vi "Create Ribbon.vi"(6 "Draw Mode":T7(ring)=enum."Triangles", 7 "3D Ribbon Property":T1={"General Property"={"Plot Name"="", "Coordinate System"=enum."Cartesian", "Opacity"=0.0}, "Projection Property"={"Draw XY"=FALSE, "Draw YZ"=FALSE, "Draw XZ"=FALSE}, "Plot Property"={"Draw Surface"=FALSE, "Color Ramp Cluster"={"Color Ramp Style"=enum."None", "Color Ramp Array"=[16711934, 393471, 57855, 4390754, 16449346, 16744722, 16711680], "Color Ramp Index"=[45, 91, 133, 175, 219, 255], "Interpolate?"=FALSE, "Logarithm?"=FALSE}, "Line Style"=enum."None", "Line Width"=0.0, "Line Color"=0, "Antialiasing"=FALSE}, "Ribbon Property"={"Ribbon Mode"=enum."Row", "Ribbon Width"=0.0}}, 8 "error in (no error)":errorcluster, 10 "Plot Representation In":T4, 11 "Plot Object In":refnum<vi>) -> (0 "error out":errorcluster, 2 "Plot Representation Out":T4, 3 "Plot Object Out":refnum<vi>, 4 "Ribbon Object Out":refnum<vi>)   [LabVIEW 2020, in "3D Ribbon.lvclass"]
uses:
  <vilib>/Math Plots/3D Math Plots/3D Ribbon/3D Ribbon/3D Ribbon.lvclass
  <vilib>/Math Plots/3D Math Plots/3D Plot/3D Plot/Typedef/Plot Representation.ctl
  <vilib>/Math Plots/3D Math Plots/3D Plot/3D Plot/Typedef/Range Clusters.ctl
  <vilib>/Math Plots/3D Math Plots/3D Plot/3D Plot/Typedef/Mesh Data.ctl
  <vilib>/Math Plots/3D Math Plots/3D Ribbon/3D Ribbon/Typedef/3D Ribbon Property.ctl
  <vilib>/Math Plots/3D Math Plots/3D Plot/3D Plot/Typedef/Color Ramp Cluster.ctl
  <vilib>/Math Plots/3D Math Plots/3D Plot/3D Plot/Typedef/Line Type.ctl
  <vilib>/picture/3D Picture Control/NI_3D Picture Control.lvlib
  <vilib>/Math Plots/3D Math Plots/3D Plot/3D Plot/3D Plot.lvclass
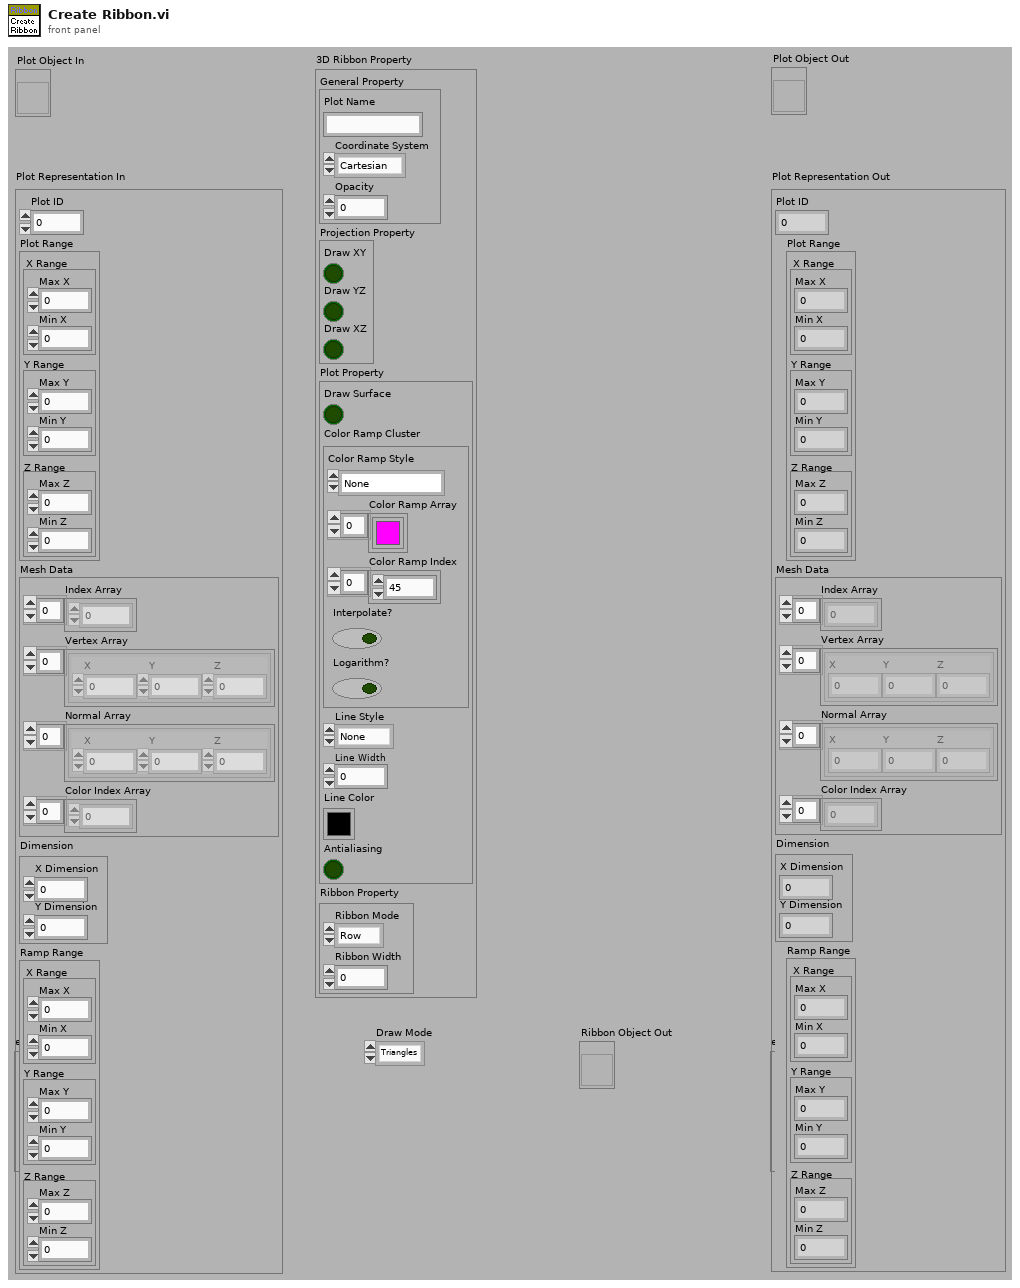
[diagram p1: front panel]
types:
  T1 = typedef "3D Ribbon.lvclass/3D Ribbon Property.ctl" = cluster{"General Property":cluster{"Plot Name":string, "Coordinate System":enum16{"Cartesian", "Cylindrical", "Spherical"}, "Opacity":sgl}, "Projection Property":cluster{"Draw XY":bool, "Draw YZ":bool, "Draw XZ":bool}, "Plot Property":cluster{"Draw Surface":bool, "Color Ramp Cluster":T2, "Line Style":T3, "Line Width":sgl, "Line Color":u32, "Antialiasing":bool}, "Ribbon Property":cluster{"Ribbon Mode":enum16{"Row", "Column"}, "Ribbon Width":sgl}}
  T2 = typedef "3D Plot.lvclass/Color Ramp Cluster.ctl" = cluster{"Color Ramp Style":enum16{"None", "Shaded", "Color spectrum", "Grey scale", "Custom"}, "Color Ramp Array":u32[], "Color Ramp Index":i32[], "Interpolate?":bool, "Logarithm?":bool}
  T3 = typedef "3D Plot.lvclass/Line Type.ctl" = enum16{"None", "Solid", "Dash", "Dot", "Dash Dot"}
  T4 = typedef "3D Plot.lvclass/Plot Representation.ctl" = cluster{"Plot ID":i32, "Plot Range":T5, "Mesh Data":T6, "Dimension":cluster{"X Dimension":i32, "Y Dimension":i32}, "Ramp Range":T5}
  T5 = typedef "3D Plot.lvclass/Range Clusters.ctl" = cluster{"X Range":cluster{"Max X":sgl, "Min X":sgl}, "Y Range":cluster{"Max Y":sgl, "Min Y":sgl}, "Z Range":cluster{"Max Z":sgl, "Min Z":sgl}}
  T6 = typedef "3D Plot.lvclass/Mesh Data.ctl" = cluster{"Index Array":u32[], "Vertex Array":cluster{"X":sgl, "Y":sgl, "Z":sgl}[], "Normal Array":cluster{"X":sgl, "Y":sgl, "Z":sgl}[], "Color Index Array":i32[]}
  T7 = enum16{"Points", "Lines", "Line Strip", "Line Loop", "Triangles", "Triangle Strip", "Triangle Fan", "Quads", "Quad Strip", "Polygon"}
  T8 = enum16{"Overall", "Per Primitive", "Per Vertex", "Binding Off"}
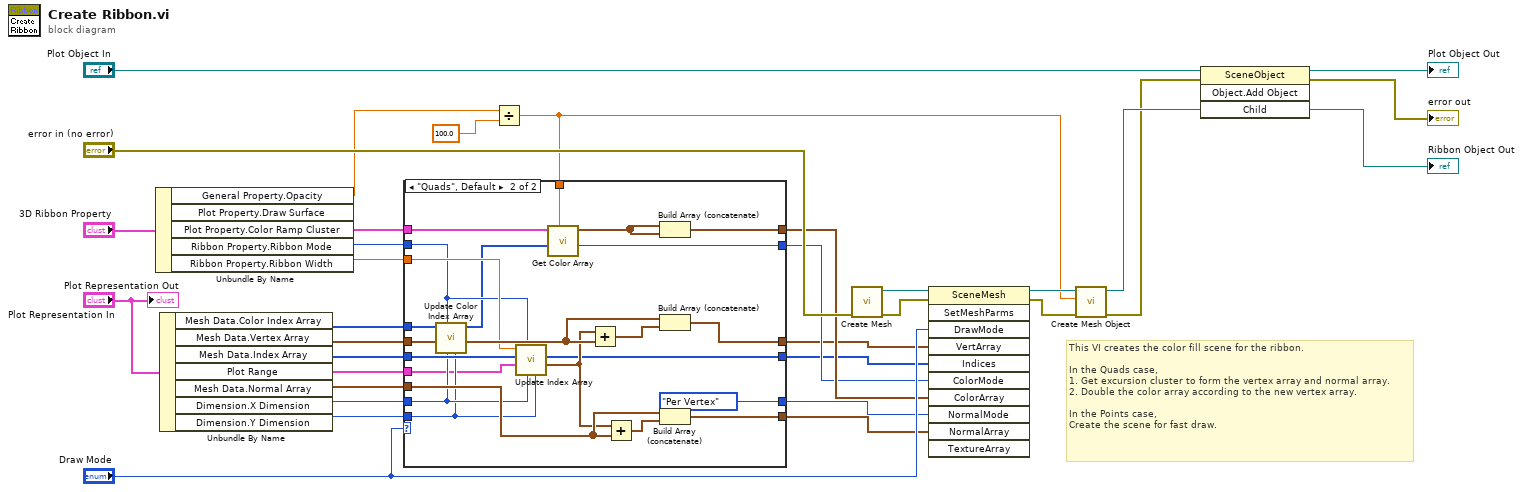
[diagram p0: block diagram]
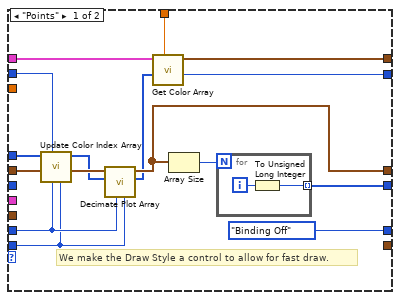
[diagram p2: hidden frame]
diagram:
  # "This VI creates the color fill scene for the ribbon.\n\nIn the Quads case, \n1. Get excursion cluster to form the vertex array and normal array.\n2. Double the color array according to the new vertex array.\n\nIn the Points case,\nCreate the scene for fast draw."
  n1 = Unbundle By Name("3D Ribbon Property") -> ("General Property.Opacity"=w14:sgl, "Plot Property.Color Ramp Cluster"=w13:T2, "Ribbon Property.Ribbon Mode"=w12:enum16{"Row", "Column"}, "Ribbon Property.Ribbon Width"=w16:sgl)  [unwired: 1 out]
  n2 = Unbundle By Name("Plot Representation In") -> ("Mesh Data.Color Index Array"=w15:i32[], "Mesh Data.Vertex Array"=w26:cluster{"X":sgl, "Y":sgl, "Z":sgl}[], "Mesh Data.Index Array"=w25:u32[], "Plot Range"=w6:T5, "Mesh Data.Normal Array"=w24:cluster{"X":sgl, "Y":sgl, "Z":sgl}[], "Dimension.X Dimension"=w22:i32, "Dimension.Y Dimension"=w21:i32)
  n3 = Divide(x=w14, y=sgl 100.0) -> (x/y=w5:sgl)
  n4 = case shown="\"Quads\", Default" "Draw Mode" {
    tunnel: w26 -> [w47 w70]
    tunnel: [w46 w71] -> w3
    tunnel: w25 -> [_ w64]
    tunnel: [w36 w54] -> w4
    tunnel: w24 -> [_ w67]
    tunnel: [_ w66] -> w2
    tunnel: w22 -> [w40 w58]
    tunnel: w21 -> [w39 w57]
    tunnel: [w45 w62] -> w19
    tunnel: [w44 w61] -> w18
    tunnel: w12 -> [w41 w56]
    tunnel: w16 -> [_ w68]
    tunnel: w15 -> [w42 w59]
    tunnel: w13 -> [w35 w52]
    tunnel: w5 -> [w43 w60]
    tunnel: w6 -> [_ w53]
    tunnel: [T8."Binding Off" ("Normal Binding Mode") T8."Per Vertex" ("Normal Binding Mode")] -> w1
    frame "Points" {
      # "We make the Draw Style a control to allow for fast draw."
      n5 = call <vilib>:"Update Color Index Array.vi"("Y Dimension"=w39, "X Dimension"=w40, "Ribbon Mode"=w41, "Color Index Array In"=w42) -> ("Color Index Array Out"=w38:i32[])  [unwired: 7 out]
      n6 = call <vilib>:"Decimate Plot Array.vi"("Y Dimension"=w39, "X Dimension"=w40, "Color Index Array In"=w38, "Vertex Array In"=w47) -> ("Color Index Array Out"=w37:i32[], "Vertex Array Out"=w46:cluster{"X":sgl, "Y":sgl, "Z":sgl}[])  [unwired: 1 in, 5 out]
      n7 = call <vilib>:"Get Color Array.vi"("Alpha"=w43, "Color Index Array"=w37, "Color Ramp Cluster"=w35) -> ("Color Binding Mode"=w44:T8, "Color Array"=w45:cluster{"R":sgl, "G":sgl, "B":sgl, "A":sgl}[])  [unwired: 4 in, 3 out]
      n8 = Array Size(array=w46) -> (size(s)=w48:i32)
      n9 = for {
        N: w48 -> [_]
        tunnel: [w49] -> w36 mode=indexing
        i -> [w50]
        n10 = To Unsigned Long Integer(number=w50) -> (unsigned 32bit integer=w49:u32)
      }
    }
    frame "Quads", Default {
      n11 = call <vilib>:"Update Color Index Array.vi"("Y Dimension"=w57, "X Dimension"=w58, "Ribbon Mode"=w56, "Color Index Array In"=w59) -> ("Color Index Array Out"=w55:i32[])  [unwired: 7 out]
      n12 = call <vilib>:"Update Index Array.vi"("Y Dimension"=w57, "X Dimension"=w58, "Ribbon Mode"=w56, "Plot Range"=w53, "Index Array Input"=w64, "Ribbon Width"=w68) -> ("Point Offset"=w65:cluster{"X":sgl, "Y":sgl, "Z":sgl}, "Index Array Output"=w54:u32[])  [unwired: 2 in, 2 out]
      n13 = call <vilib>:"Get Color Array.vi"("Alpha"=w60, "Color Index Array"=w55, "Color Ramp Cluster"=w52) -> ("Color Binding Mode"=w61:T8, "Color Array"=w63:cluster{"R":sgl, "G":sgl, "B":sgl, "A":sgl}[])  [unwired: 4 in, 3 out]
      n14 = Add(x=w65, y=w70) -> (x+y=w72:cluster{"X":sgl, "Y":sgl, "Z":sgl}[])
      n15 = Add(x=w65, y=w67) -> (x+y=w69:cluster{"X":sgl, "Y":sgl, "Z":sgl}[])
      n16 = Build Array (concatenate)(w63, w63) -> (w62:cluster{"R":sgl, "G":sgl, "B":sgl, "A":sgl}[])
      n17 = Build Array (concatenate)(w70, w72) -> (w71:cluster{"X":sgl, "Y":sgl, "Z":sgl}[])
      n18 = Build Array (concatenate)(w67, w69) -> (w66:cluster{"X":sgl, "Y":sgl, "Z":sgl}[])
    }
  }
  n19 = call <vilib>:"Create Mesh.vi"("error in (no error)"="error in (no error)") -> ("error out"=w23:errorcluster, "New Mesh Refnum"=w27:refnum<vi>)  [unwired: 9 out]
  n20 = invoke class="SceneMesh" method="SetMeshParms"(reference=w27, error in=w23, "DrawMode"="Draw Mode", "VertArray"=w3, "Indices"=w4, "ColorMode"=w18, "ColorArray"=w19, "NormalMode"=w1, "NormalArray"=w2) -> (reference out=w11:refnum<vi>, error out=w10:errorcluster)  [unwired: 2 in, 9 out]
  n21 = call <vilib>:"Create Mesh Object.vi"("error in (no error)"=w10, "Alpha"=w5, "Mesh Object In"=w11) -> ("error out"=w8:errorcluster, "Object Ref Out"=w9:refnum<vi>)  [unwired: 1 in, 6 out]
  n22 = invoke class="SceneObject" method="Object.Add Object"(reference="Plot Object In", error in=w8, "Child"=w9) -> (reference out=→"Plot Object Out":refnum<vi>, error out=→"error out":errorcluster, "Child"=→"Ribbon Object Out":refnum<vi>)  [unwired: 1 in, 1 out]
  "Plot Representation Out" <- "Plot Representation In"
